vi "sub vi - save log dir V1.vi"(11 "Dir Input":string) -> ()   [LabVIEW 2013]
uses:
  program files/Global 1.vi
panel:
  out "error out":errorcluster
  out "network dir":string
  out "file dir":string
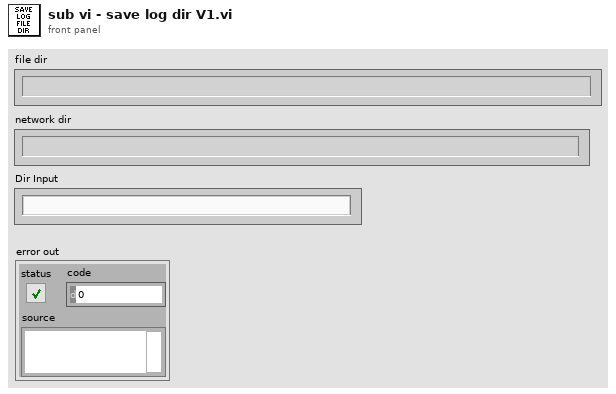
[diagram p1: front panel]
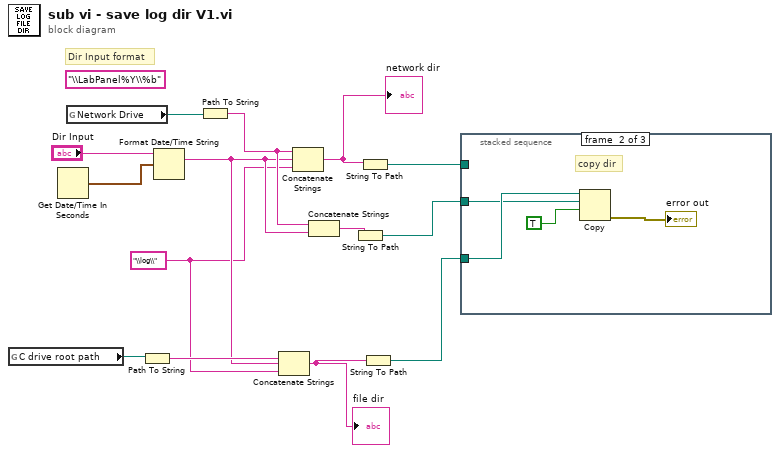
[diagram p0: block diagram]
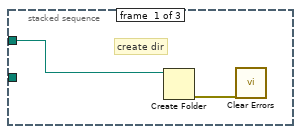
[diagram p2: hidden frame]
diagram:
  w1 = "\\log\\"
  (unwired) "\\LabPanel%Y\\%b"
  # "Dir Input format"
  n1 = global read "Global 1.vi" "C drive root path"() -> (w11:path)
  n2 = Get Date/Time In Seconds() -> (seconds since 1Jan1904=w13:timestamp)
  n3 = global read "Global 1.vi" "Network Drive"() -> (w14:path)
  n4 = Path To String(path=w11) -> (string=w12:string)
  n5 = Format Date/Time String(time format string (%c)="Dir Input", seconds (now)=w13) -> (date/time string=w5:string)  [unwired: 1 in]
  n6 = Path To String(path=w14) -> (string=w6:string)
  n7 = Concatenate Strings(w12, w5, w1) -> (w9:string)
  "file dir" <- w9
  n8 = Concatenate Strings(w6, w5, w1) -> (w10:string)
  "network dir" <- w10
  n9 = Concatenate Strings(w6, w5) -> (w4:string)
  n10 = String To Path(string=w4) -> (path=w3:path)
  n11 = String To Path(string=w10) -> (path=w8:path)
  n12 = String To Path(string=w9) -> (path=w7:path)
  n13 = stacked-sequence {
    tunnel: w8 -> [w15 _ _]
    tunnel: w7 -> [_ w19 _]
    tunnel: w3 -> [_ w17 _]
    frame #0 {
      # "create dir"
      n14 = Create Folder(path (use dialog)=w15) -> (error out=w16:errorcluster)  [unwired: 2 in, 2 out]
      n15 = call <vilib>:"Clear Errors.vi"("error in (no error)"=w16) -> ()  [unwired: 6 in, 1 out]
    }
    frame #1 {
      # "copy dir"
      n16 = Copy(9:TRUE, 10:w17, 11:w19) -> (0:→"error out":errorcluster)  [unwired: 2 in, 2 out]
    }
    frame #2 {
    }
  }
